vi "Status.vi"(8 "error in (no error)":errorcluster, 10 "Internal?":bool, 11 "Huber Settings In":T1) -> (0 "error out":errorcluster, 1 "Connection Error":bool, 2 "Running":bool, 3 "Huber Settings Out":T1, 6 "Temperature":dbl)   [LabVIEW 2021, in "Huber Unistat 410 TCU.lvlib"]
uses:
  Huber Unistat 410 TCU.lvlib
  Huber Unistat 410 Settings.ctl
  <vilib>/regexp/Match Regular Expression.xnode
panel:
  out "substring":string
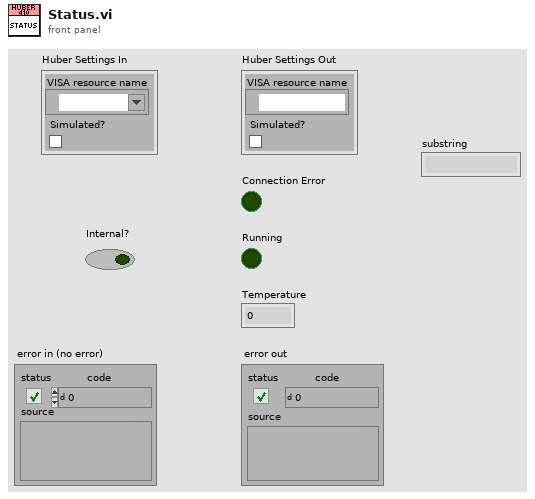
[diagram p1: front panel]
types:
  T1 = typedef "Huber Unistat 410 TCU.lvlib/Huber Unistat 410 Settings.ctl" = cluster{"VISA resource name":refnum<visa-resource-name>, "Simulated?":bool}
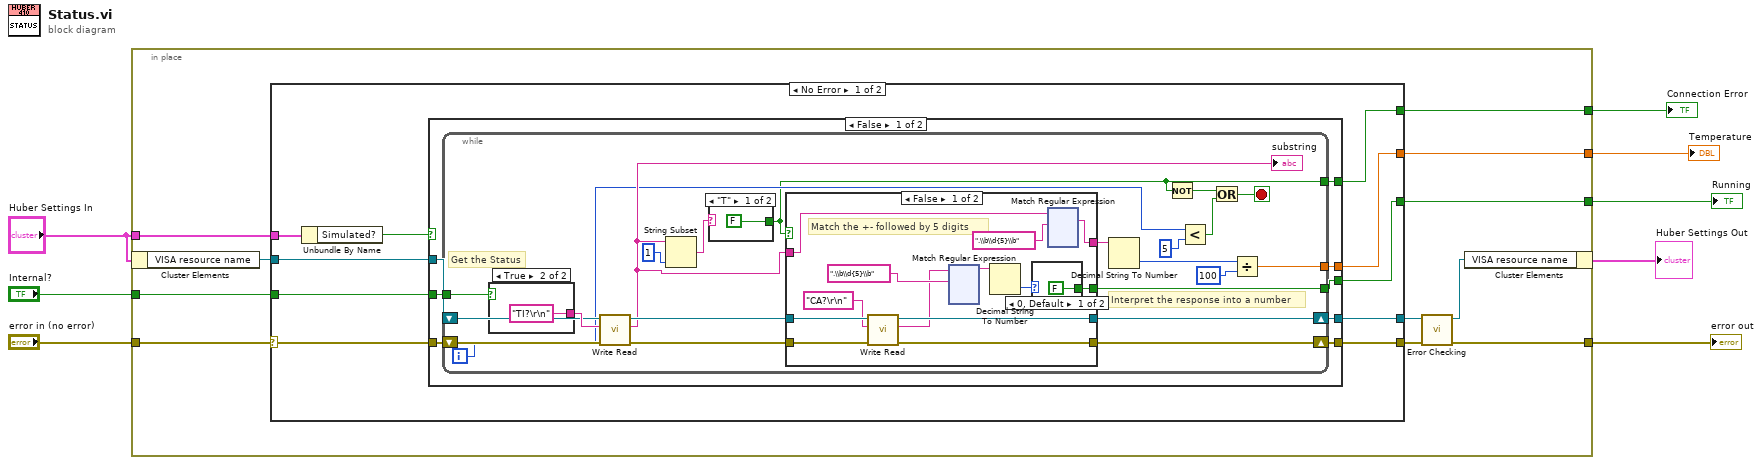
[diagram p0: block diagram]
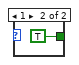
[diagram p2: hidden frame]
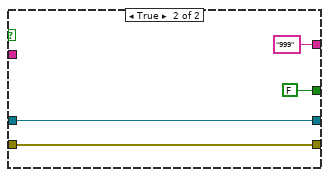
[diagram p3: hidden frame]
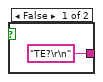
[diagram p4: hidden frame]
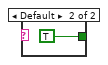
[diagram p5: hidden frame]
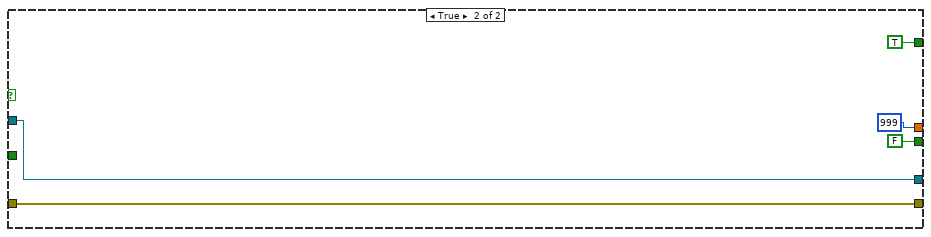
[diagram p6: hidden frame]
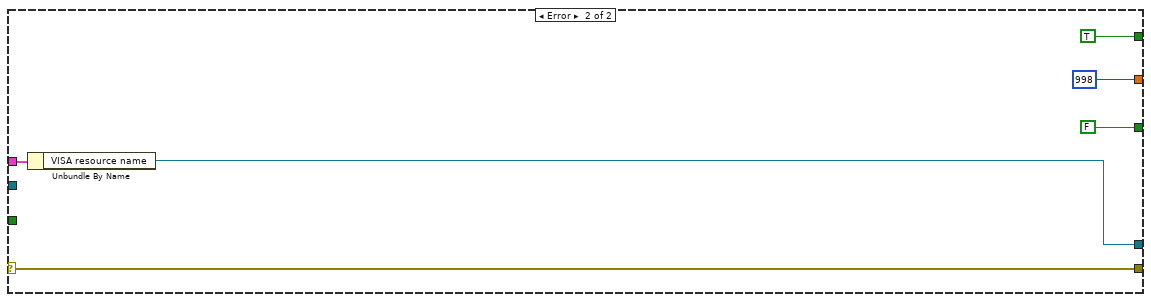
[diagram p7: hidden frame]
diagram:
  n1 = in-place {
    in-place-border: "error in (no error)" -> [w19]
    in-place-border: [w16] -> w7
    in-place-border: "Huber Settings In" -> [w15]
    in-place-border: [w14] -> w6
    in-place-border: [w13] -> w5
    in-place-border: [w12] -> w4
    in-place-border: "Internal?" -> [w11]
    n2 = in-place-cluster #1("Huber Settings In") -> ("VISA resource name"=w10:refnum<visa-resource-name>)
    n3 = case shown="No Error" w19 {
      selector: w19 -> [w29 w327]
      tunnel: w15 -> [w27 w326]
      tunnel: [w28 w327] -> w17
      tunnel: [w26 w325] -> w18
      tunnel: [w24 TRUE] -> w14
      tunnel: [w23 FALSE] -> w13
      tunnel: [w22 998] -> w12
      tunnel: w11 -> [w21 _]
      tunnel: w10 -> [w20 _]
      frame No Error {
        n4 = Unbundle By Name(w27) -> ("Simulated?"=w25:bool)
        n5 = case shown="False" w25 {
          tunnel: w29 -> [w36 w321]
          tunnel: [w34 w321] -> w28
          tunnel: [w32 w320] -> w26
          tunnel: w20 -> [w37 w320]
          tunnel: [w35 TRUE] -> w24
          tunnel: [w33 FALSE] -> w23
          tunnel: [w30 999] -> w22
          tunnel: w21 -> [w31 _]
          frame False {
            n6 = while {
              tunnel: [w39] -> w35
              tunnel: [w51] -> w33
              tunnel: w31 -> [w48]
              tunnel: [w45] -> w30
              shift-right: [w50] -> w32
              shift-left: w37 -> [w57]
              shift-right: [w53] -> w34
              shift-left: w36 -> [w56]
              i -> [w40]
              stop <- w38 stop-if-true
              # "Interpret the response into a number"
              # "Get the Status"
              n7 = case shown="True" w48 {
                tunnel: ["TE?\r\n" ("string") "TI?\r\n" ("string")] -> w59
                frame False {
                }
                frame True {
                }
              }
              n8 = call "Write Read.vi"("error in (no error)"=w56, "write string"=w59, "VISA Refnum in"=w57) -> ("error out"=w54:errorcluster, "read string"=w47:string, "VISA Refnum out"=w52:refnum<visa-resource-name>)  [unwired: 6 in]
              "substring" <- w47
              n9 = String Subset(string=w47, length (rest)=1 ("length (rest)")) -> (substring=w55:string)  [unwired: 1 in]
              n10 = case shown="\"T\"" w55 {
                tunnel: [FALSE TRUE] -> w39
                frame "T" {
                }
                frame Default {
                }
              }
              n11 = case shown="False" w39 {
                tunnel: w47 -> [w72 _]
                tunnel: [w71 "999" ("whole match")] -> w49
                tunnel: w54 -> [w65 w311]
                tunnel: [w64 w311] -> w53
                tunnel: w52 -> [w67 w309]
                tunnel: [w69 FALSE] -> w51
                tunnel: [w63 w309] -> w50
                frame False {
                  # "Match the +- followed by 5 digits"
                  n12 = call "Write Read.vi"("error in (no error)"=w65, "write string"="CA?\r\n" ("string"), "VISA Refnum in"=w67) -> ("error out"=w64:errorcluster, "read string"=w61:string, "VISA Refnum out"=w63:refnum<visa-resource-name>)  [unwired: 6 in]
                  n13 = xnode "Match Regular Expression"("input string"=w61, "regular expression"=".\\b\\d{5}\\b") -> ("whole match"=w60:string)  [unwired: 4 in, 4 out]
                  n14 = Decimal String To Number(string=w60) -> (number=w68:i32)  [unwired: 2 in, 1 out]
                  n15 = case shown="0, Default" w68 {
                    tunnel: [FALSE TRUE] -> w69
                    frame 0, Default {
                    }
                    frame 1 {
                    }
                  }
                  n16 = xnode "Match Regular Expression"("input string"=w72, "regular expression"=".\\b\\d{5}\\b") -> ("whole match"=w71:string)  [unwired: 4 in, 4 out]
                }
                frame True {
                }
              }
              n17 = Decimal String To Number(string=w49) -> (number=w46:i32)  [unwired: 2 in, 1 out]
              n18 = Not(x=w39) -> (.not. x?=w42:bool)
              n19 = Less?(x=w40, y=5) -> (x < y?=w41:bool)
              n20 = Or(x=w42, y=w41) -> (x .or. y?=w38:bool)
              n21 = Divide(x=w46, y=100) -> (x/y=w45:dbl)
            }
          }
          frame True {
          }
        }
      }
      frame Error {
        n22 = Unbundle By Name(w326) -> ("VISA resource name"=w325:refnum<visa-resource-name>)
      }
    }
    n23 = call "Error Checking.vi"("error in (no error)"=w17, "VISA resource name"=w18) -> ("error out"=w16:errorcluster, "VISA resource name"=w9:refnum<visa-resource-name>)  [unwired: 7 in, 1 out]
    n24 = in-place-cluster #1("VISA resource name"=w9) -> (→"Huber Settings Out":T1)
  }
  "error out" <- w7
  "Connection Error" <- w6
  "Running" <- w5
  "Temperature" <- w4
